vi "Fire Do Turn Event.vi"(8 "error in (no error)":errorcluster, 10 "Single Step":bool, 11 "SB App in":refnum<class "SB App.lvclass">) -> (0 "error out":errorcluster)   [LabVIEW 2020, in "SB App.lvlib" / "SB App.lvclass"]
uses:
  SB App.lvclass
  SB App.lvclass/SB App.ctl
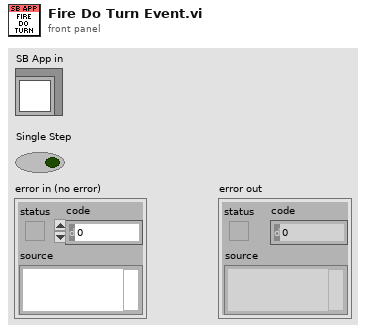
[diagram p1: front panel]
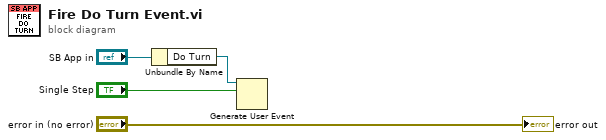
[diagram p0: block diagram]
diagram:
  n1 = Unbundle By Name("SB App in") -> ("Do Turn"=w2:refnum<user-event>)
  n2 = Generate User Event(user event=w2, event data cluster="Single Step") -> ()  [unwired: 2 in, 2 out]
  "error out" <- "error in (no error)"
